vi "Rinocloud_HTTP_metadata_to_tree.vi"(8 "error in (no error)":errorcluster, 10 "JSON Tree Expanded Reference":refnum<vi>, 11 "id":string) -> (0 "error out":errorcluster, 1 "Notes":string, 2 "Tags":string, 3 "Name":string, 4 "Status":T1={"headers"="", "body"="", "ID"="", "Saved"=TRUE}, 5 "metadata (JSON)":string)   [LabVIEW 2011, in "Rinocloud Library.lvlib"]
uses:
  Rinocloud Library.lvlib
  i3 JSON/i3-json.lvlib
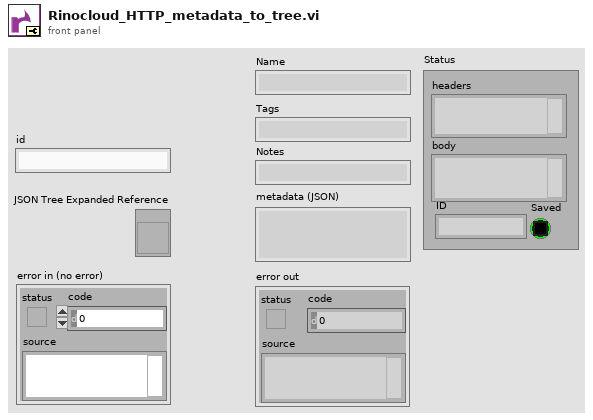
[diagram p1: front panel]
types:
  T1 = cluster{"headers":string, "body":string, "ID":string, "Saved":bool}
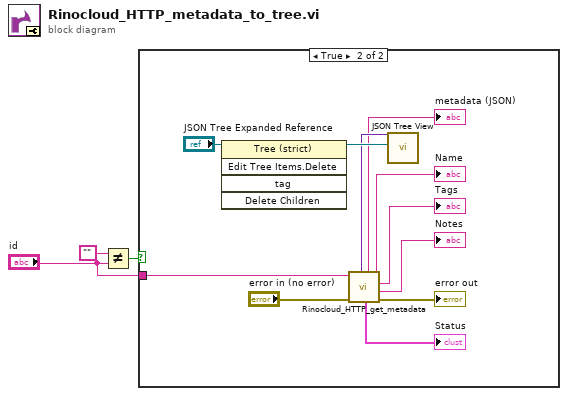
[diagram p0: block diagram]
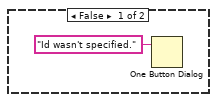
[diagram p2: hidden frame]
diagram:
  n1 = Not Equal?(x="", y="id") -> (x != y?=w2:bool)
  n2 = case shown="True" w2 {
    tunnel: "id" -> [_ w7]
    frame False {
      n3 = One Button Dialog(message="Id wasn't specified.") -> ()  [unwired: 1 in, 1 out]
    }
    frame True {
      n4 = invoke class="Tree (strict)" method="Edit Tree Items.Delete"(reference="JSON Tree Expanded Reference") -> (reference out=w14:refnum<vi>)  [unwired: 4 in, 4 out]
      n5 = call "Rinocloud_HTTP_get_metadata.vi"("error in (no error)"="error in (no error)", "id"=w7) -> ("error out"=→"error out":errorcluster, "Notes"=→"Notes":string, "Tags"=→"Tags":string, "Name"=→"Name":string, "Status"=→"Status":T1, "metadata (JSON)"=→"metadata (JSON)":string, "JSON Object"=w13:variant)  [unwired: 3 in]
      n6 = call "JSON Tree View.vi"("JSON Tree Expanded Reference"=w14, "JSON Tree"=w13) -> ()  [unwired: 8 in, 2 out]
    }
  }
